vi "find_spectrometers.vi"(8 "error in (no error)":errorcluster, 11 "UV-VIS_AVANTES in":refnum<class "UV-VIS_AVANTES.lvclass">) -> (0 "error out":errorcluster, 2 "List Output":u8[](array[numeric]), 3 "UV-VIS_AVANTES out":refnum<class "UV-VIS_AVANTES.lvclass">)   [LabVIEW 2019, in "UV-VIS_AVANTES.lvclass"]
uses:
  UV-VIS_AVANTES.lvclass
  UV-VIS_AVANTES.lvclass/UV-VIS_AVANTES.ctl
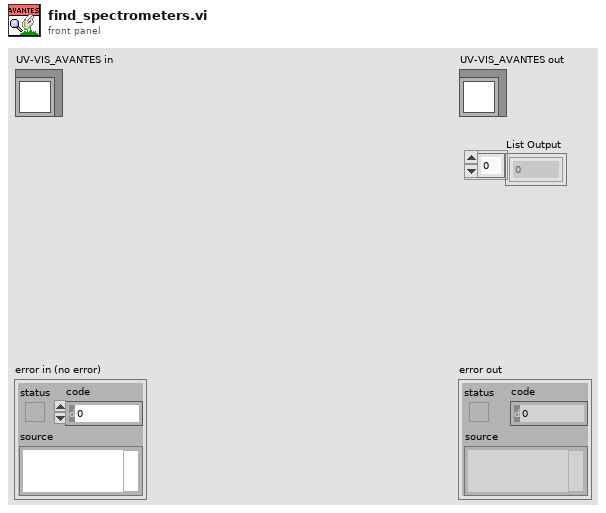
[diagram p1: front panel]
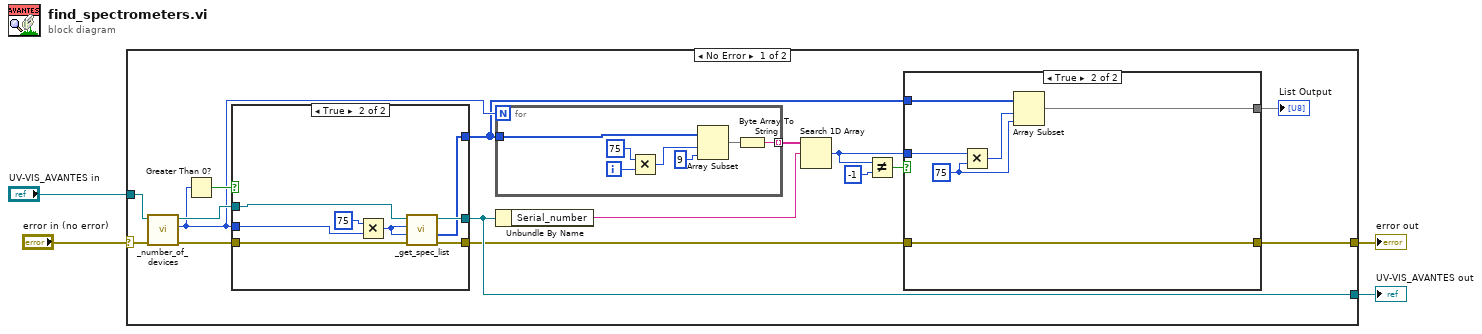
[diagram p0: block diagram]
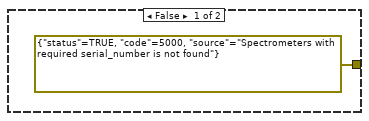
[diagram p2: hidden frame]
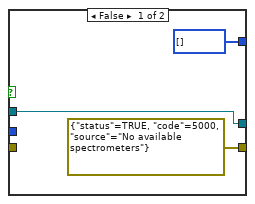
[diagram p3: hidden frame]
diagram:
  n1 = case shown="No Error" "error in (no error)" {
    selector: "error in (no error)" -> [w19 w47]
    tunnel: [w13 w46] -> w2
    tunnel: "UV-VIS_AVANTES in" -> [w20 w46]
    tunnel: [w5 w47] -> w1
    frame No Error {
      n2 = call "_number_of_devices.vi"("error in (no error)"=w19, "UV-VIS_AVANTES in"=w20) -> ("error out"=w17:errorcluster, "# spectrometers"=w15:i32, "UV-VIS_AVANTES out"=w18:refnum<class "UV-VIS_AVANTES.lvclass">)  [unwired: 7 in]
      n3 = Greater Than 0?(x=w15) -> (x > 0?=w16:bool)
      n4 = case shown="True" w16 {
        tunnel: w18 -> [w35 w45]
        tunnel: [w35 w44] -> w13
        tunnel: [errorcluster {"status"=TRUE, "code"=5000, "source"="No available spectrometers"} ("error out") w43] -> w6
        tunnel: w17 -> [_ w42]
        tunnel: [u8[] [] w41] -> w8
        tunnel: w15 -> [_ w38]
        frame False {
        }
        frame True {
          n5 = Multiply(x=75, y=w38) -> (x*y=w39:i32)
          n6 = call "_get_spec_list.vi"("error in (no error)"=w42, "RequiredSizeInput"=w39, "ListSizeInput"=w39, "UV-VIS_AVANTES in"=w45) -> ("error out"=w43:errorcluster, "List Output"=w41:u8[], "UV-VIS_AVANTES out"=w44:refnum<class "UV-VIS_AVANTES.lvclass">)  [unwired: 5 in]
        }
      }
      n7 = for {
        N: w15 -> [_]
        tunnel: w8 -> [w29]
        tunnel: [w28] -> w14 mode=indexing
        i -> [w30]
        n8 = Multiply(x=75, y=w30) -> (x*y=w33:i32)
        n9 = Array Subset(array=w29, index=w33, length=9) -> (w34:u8[])
        n10 = Byte Array To String(unsigned byte array=w34) -> (string=w28:string)
      }
      n11 = Unbundle By Name(w13) -> ("Serial_number"=w12:string)
      n12 = Search 1D Array(1D array=w14, element=w12) -> (index of element=w9:i32)  [unwired: 1 in]
      n13 = Not Equal?(x=w9, y=-1) -> (x != y?=w10:bool)
      n14 = case shown="True" w10 {
        tunnel: w9 -> [_ w27]
        tunnel: w8 -> [_ w26]
        tunnel: [_ w23] -> w7
        tunnel: w6 -> [_ w22]
        tunnel: [errorcluster {"status"=TRUE, "code"=5000, "source"="Spectrometers with required serial_number is not found"} ("error out") w22] -> w5
        frame False {
        }
        frame True {
          w24 = 75 ("y")
          n15 = Multiply(x=w27, y=w24) -> (x*y=w25:i32)
          n16 = Array Subset(array=w26, index=w25, length=w24) -> (w23:u8[])
        }
      }
      "List Output" <- w7
    }
    frame Error {
    }
  }
  "error out" <- w1
  "UV-VIS_AVANTES out" <- w2
